vi "DriveStraightDistanceNavX.vi"(0 "Time":dbl=5.0 caption="Time Target (s)", 1 "Lift":dbl format="%#_13g", 4 "LiftMode":bool=TRUE, 5 "Speed":dbl=0.4 format="%#_13g", 6 "WristMode":bool=TRUE, 7 "Angle":dbl, 9 "Distance":dbl=5.0 format="%#_13g", 11 "Wrist":dbl format="%#_13g", 12 "Intake":dbl format="%#_13g") -> ()   [LabVIEW 2017]
uses:
  Phoenix-LabVIEW/Motor Controller/Controls/CTRE_Phoenix_MotorControl_ControlMode.ctl
  Robot Global Data.vi
  <vilib>/addons/control/pid/pid.llb/PID (DBL).vi
  <vilib>/addons/control/pid/NI_PID_pid.lvlib
panel:
  in  "Encoders":T1={"proportional gain (Kc)"=0.015, "integral time (Ti, min)"=0.0, "derivative time (Td, min)"=0.0} {"derivative time (Td, min)" format="%.3f"; "integral time (Ti, min)" format="%.3f"; "proportional gain (Kc)" format="%.3f"}
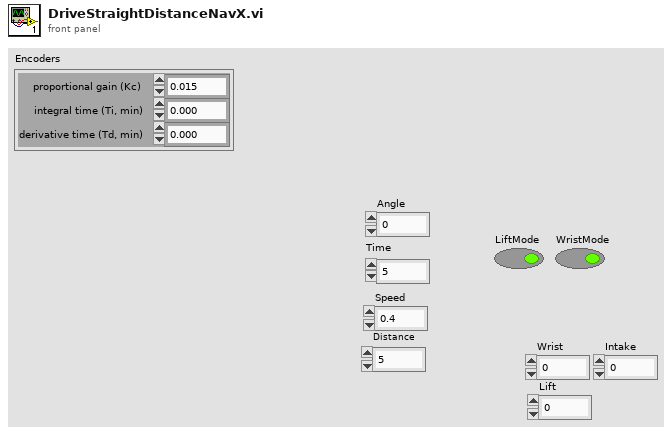
[diagram p1: front panel]
types:
  T1 = cluster{"proportional gain (Kc)":dbl, "integral time (Ti, min)":dbl, "derivative time (Td, min)":dbl}
  T2 = typedef "CTRE_Phoenix_MotorControl_ControlMode.ctl" = u16
  T3 = typedef "WPI_MotorControlDeviceRef.ctl" = cluster{"DeviceStatus":errorcluster, "Type":T4, "PWM":cluster{"PWM Channel":T5, "DeadBand":T6}, "CAN":cluster{"Device Number":u8, "SetOutput VI Ref":variant, "GetOutput VI Ref":variant, "Enable VI Ref":variant, "Disable VI Ref":variant, "Data":variant}, "Invert":bool, "DIO PWM":cluster{"PWM \"Enable\" Channel":T5, "DIOChannel":T7, "PWM Rate":dbl}}
  T4 = typedef "WPI_MotorControlType.ctl" = enum16{"PWM", "CAN", "DIO PWM"}
  T5 = typedef "FPGA_DIOPWMChannel.ctl" = enum8{"PWM 0", "PWM 1", "PWM 2", "PWM 3", "PWM 4", "PWM 5", "PWM 6", "PWM 7", "PWM 8", "PWM 9", "PWM MXP 0", "PWM MXP 1", "PWM MXP 2", "PWM MXP 3", "PWM MXP 4", "PWM MXP 5", "PWM MXP 6", "PWM MXP 7", "PWM MXP 8", "PWM MXP 9", "Invalid"}
  T6 = typedef "WPI_PWMDeadband.ctl" = cluster{"Name":string, "maxPositivePwm":i32, "minPositivePwm":i32, "centerPwm":i32, "maxNegativePwm":i32, "minNegativePwm":i32, "angularRange":u16}
  T7 = typedef "FPGA_DIOChannel.ctl" = enum8{"DIO 0", "DIO 1", "DIO 2", "DIO 3", "DIO 4", "DIO 5", "DIO 6", "DIO 7", "DIO 8", "DIO 9", "DIO MXP 0", "DIO MXP 1", "DIO MXP 2", "DIO MXP 3", "DIO MXP 4", "DIO MXP 5", "DIO MXP 6", "DIO MXP 7", "DIO MXP 8", "DIO MXP 9", "DIO MXP 10", "DIO MXP 11", "DIO MXP 12", "DIO MXP 13", "DIO MXP 14", "DIO MXP 15", "SPI Port CS1", "SPI Port CS2", "SPI Port CS3", "SPI Port MISO", "SPI Port MOSI", "Invalid"}
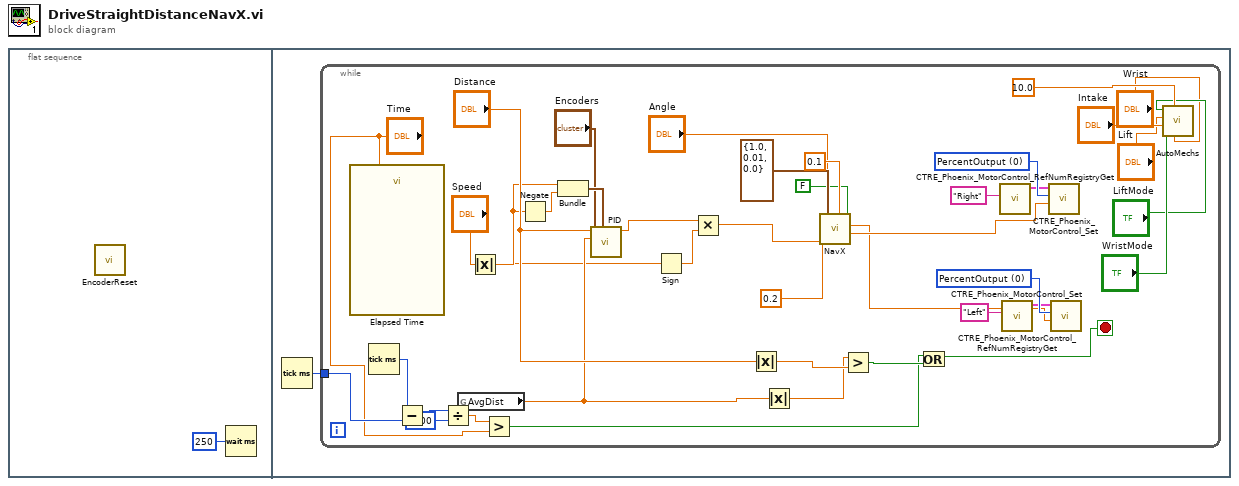
[diagram p0: block diagram]
diagram:
  n1 = flat-sequence {
    frame #0 {
      n2 = call "EncoderReset.vi"() -> ()  [unwired: 12 in]
      n3 = Wait (ms)(milliseconds to wait=u32 250) -> ()  [unwired: 1 out]
    }
    frame #1 {
      n4 = Tick Count (ms)() -> (millisecond timer value=w2:u32)
      n5 = while {
        tunnel: w2 -> [w12]
        stop <- w29 stop-if-true
        w36 = T2 0 items=["PercentOutput"=0, "Position"=1, "Velocity"=2, "Current"=3, "Follower"=5, "MotionProfile"=6, "MotionMagic"=7, "MotionMagicArc"=8, "MotionProfileArc"=10, "Disabled"=15] ("Control Mode")
        w39 = T2 0 items=["PercentOutput"=0, "Position"=1, "Velocity"=2, "Current"=3, "Follower"=5, "MotionProfile"=6, "MotionMagic"=7, "MotionMagicArc"=8, "MotionProfileArc"=10, "Disabled"=15] ("Control Mode")
        n6 = call "Elapsed Time"("Time Target (s)"="Time") -> ()  [unwired: 11 in, 8 out]
        n7 = Tick Count (ms)() -> (millisecond timer value=w13:u32)
        n8 = Subtract(x=w13, y=w12) -> (x-y=w11:u32)
        n9 = Divide(x=w11, y=u32 1000) -> (x/y=w9:dbl)
        n10 = global read "Robot Global Data.vi" "AvgDist"() -> (w24:dbl)
        n11 = Absolute Value(x="Speed") -> (abs(x)=w20:dbl)
        n12 = Greater?(x=w9, y="Time") -> (0:w7:bool)
        n13 = Negate(x=w20) -> (-x=w27:dbl)
        n14 = Bundle(w20, w27) -> (w26:cluster{dbl, dbl})  [unwired: 1 in]
        n15 = call-poly <vilib>:"PID.vi"("output range"=w26, "PID gains"="Encoders", "process variable"=w24, "setpoint"="Distance") -> ("output"=w18:dbl)  [unwired: 6 in, 1 out]
        n16 = Sign(1:"Speed") -> (0:w17:dbl)
        n17 = Multiply(x=w18, y=w17) -> (x*y=w16:dbl)
        n18 = Absolute Value(x="Distance") -> (abs(x)=w15:dbl)
        n19 = Absolute Value(x=w24) -> (abs(x)=w14:dbl)
        n20 = call "NavX.vi"("PID gains"=T1 {"proportional gain (Kc)"=1.0, "integral time (Ti, min)"=0.01, "derivative time (Td, min)"=0.0} ("PID_NAVX"), "AngleSetpoint"="Angle", "MaxSpeed"=0.2, "NavxSpeed"=w16, "NavX_P"=0.1, "PID?"=FALSE) -> ("LeftNavx"=w32:dbl, "RightNavx"=w33:dbl)  [unwired: 1 out]
        n21 = Greater?(x=w14, y=w15) -> (0:w30:bool)
        n22 = Or(x=w7, y=w30) -> (x .or. y?=w29:bool)
        n23 = call "CTRE_Phoenix_MotorControl_RefNumRegistryGet.vi"("refnum name"="Right") -> ("PhoenixMotorControlDevRef"=w35:T3)  [unwired: 9 in, 1 out]
        n24 = call "CTRE_Phoenix_MotorControl_RefNumRegistryGet.vi"("refnum name"="Left") -> ("PhoenixMotorControlDevRef"=w38:T3)  [unwired: 9 in, 1 out]
        n25 = call "CTRE_Phoenix_MotorControl_Set.vi"("Output"=w33, "Control Mode"=w36, "PhoenixMotorControlDevRef"=w35) -> ()  [unwired: 7 in, 2 out]
        n26 = call "CTRE_Phoenix_MotorControl_Set.vi"("Output"=w32, "Control Mode"=w39, "PhoenixMotorControlDevRef"=w38) -> ()  [unwired: 7 in, 2 out]
        n27 = call "AutoMechs.vi"("Wrist"="Wrist", "Time"=10.0, "WristMode"="WristMode", "Intake"="Intake", "Lift"="Lift", "LiftMode"="LiftMode") -> ()  [unwired: 6 in]
      }
    }
  }
